vi "HFRR ADV v024 new software.vi"() -> ()   [LabVIEW 2025] (continued)
    tunnel: [w2159] -> _
    tunnel: [w2135] -> w60
    i -> [w2159]
    stop <- w2135 stop-if-true
    # "C:\\LAB-IQ-NXT\\Scar View.exe"
    n1674 = local read "OK Button 16"() -> (w2148:bool)
    n1675 = local read "Main Tab"() -> (w2141:T2)
    n1676 = local read "service 3"() -> (w2142:bool)
    n1677 = local read "OPEN 6"() -> (w2144:bool)
    n1678 = local read "EDIT 2"() -> (w2146:bool)
    n1679 = flat-sequence {
      frame #0 {
        n1680 = stacked-sequence {
          frame #0 {
            n1681 = local read "EDIT"() -> (w2813:bool)
            n1682 = case shown="True" w2813 {
              tunnel: [u8 2 ("Disabled") u8 0 ("Disabled")] -> _
              frame False {
                w2815 = FALSE
                n1683 = local write "Password"("") -> ()
                n1684 = property on="SrvM CP" class="Bool (strict)"("Visible"=w2815) -> ()  [unwired: 2 in, 2 out]
                n1685 = property on="message" class="Str"("Visible"=w2815) -> ()  [unwired: 2 in, 2 out]
                n1686 = local write "x = y?"(w2815) -> ()
                n1687 = property on="Password" class="Str"("Visible"=w2815) -> ()  [unwired: 2 in, 2 out]
                n1688 = property on="ENTER THE NEW PASSWORD" class="Str"("Visible"=w2815) -> ()  [unwired: 2 in, 2 out]
                n1689 = property on="ENTER CURRENT PASSWORD" class="Str"("Visible"=w2815) -> ()  [unwired: 2 in, 2 out]
                n1690 = local write "SrvM CP"(w2815) -> ()
              }
              frame True {
                w2818 = TRUE
                n1691 = property on="SrvM CP" class="Bool (strict)"("Visible"=w2818) -> ()  [unwired: 2 in, 2 out]
                n1692 = property on="Password" class="Str"("Visible"=w2818) -> ()  [unwired: 2 in, 2 out]
              }
            }
            "dipl pwd" <- "@143$\n" ("dipl pwd")
          }
          frame #1 {
            # "Gain password"
            n1693 = String To Byte Array(string="ENTER CURRENT PASSWORD") -> (unsigned byte array=w2823:u8[])
            n1694 = Search 1D Array(1D array=w2823, element=u8 10) -> (index of element=w2826:i32)  [unwired: 1 in]
            n1695 = Index Array(array=w2823, index=w2826) -> (element=w2822:u8)
            n1696 = Equal?(x=w2822, y=10) -> (x = y?=w2820:bool)
            n1697 = case shown="True" w2820 {
              frame False {
                n1698 = property on="ENTER THE NEW PASSWORD" class="Str"("Visible"=FALSE) -> ()  [unwired: 2 in, 2 out]
              }
              frame True {
                # "password"
                # "change password logic"
                n1699 = local read "ENTER CURRENT PASSWORD"() -> (w2839:string)
                n1700 = local read "dipl pwd"() -> (w2833:string)
                n1701 = String To Byte Array(string=w2839) -> (unsigned byte array=w2841:u8[])
                n1702 = String To Byte Array(string=w2833) -> (unsigned byte array=w2834:u8[])
                n1703 = Array Size(array=w2841) -> (size(s)=w2838:i32)
                n1704 = Array Size(array=w2834) -> (size(s)=w2836:i32)
                n1705 = for {
                  N: w2838 -> [_]
                  tunnel: w2841 -> [w2865]
                  tunnel: [w2863] -> w2842 mode=indexing
                  tunnel: w2838 -> [w2857]
                  i -> [w2858]
                  n1706 = Decrement(x=w2857) -> (x-1=w2855:i32)
                  n1707 = Equal?(x=w2858, y=w2855) -> (x = y?=w2856:bool)
                  n1708 = Index Array(array=w2865, index=w2858) -> (element=w2859:u8)
                  n1709 = Number To Decimal String(number=w2859) -> (decimal integer string=w2864:string)  [unwired: 1 in]
                  n1710 = Select(t="", s=w2856, f="\r") -> (s? t:f=w2861:string)
                  n1711 = Concatenate Strings(w2864, w2861) -> (w2863:string)
                }
                n1712 = for {
                  N: w2836 -> [_]
                  tunnel: w2834 -> [w2853]
                  tunnel: [w2851] -> w2835 mode=indexing
                  tunnel: w2836 -> [w2848]
                  i -> [w2849]
                  n1713 = Decrement(x=w2848) -> (x-1=w2847:i32)
                  n1714 = Equal?(x=w2849, y=w2847) -> (x = y?=w2846:bool)
                  n1715 = Index Array(array=w2853, index=w2849) -> (element=w2852:u8)
                  n1716 = Number To Decimal String(number=w2852) -> (decimal integer string=w2850:string)  [unwired: 1 in]
                  n1717 = Select(t="", s=w2846, f="\r") -> (s? t:f=w2843:string)
                  n1718 = Concatenate Strings(w2850, w2843) -> (w2851:string)
                }
                n1719 = local read "string"() -> (w2840:string)
                n1720 = Concatenate Strings(w2835) -> (w2829:string)
                n1721 = Concatenate Strings(w2840) -> (w2837:string)
                n1722 = Concatenate Strings(w2842) -> (w2830:string)
                n1723 = Equal?(x=w2830, y=w2837) -> (x = y?=w2832:bool)
                n1724 = Equal?(x=w2830, y=w2829) -> (x = y?=w2828:bool)
                n1725 = Or(x=w2832, y=w2828) -> (x .or. y?=w2831:bool)
                n1726 = case shown="True" w2831 {
                  frame False {
                  }
                  frame True {
                    n1727 = property on="ENTER THE NEW PASSWORD" class="Str"("Visible"=TRUE) -> ()  [unwired: 2 in, 2 out]
                  }
                }
              }
            }
          }
          frame #2 {
            n1728 = String To Byte Array(string="ENTER THE NEW PASSWORD") -> (unsigned byte array=w2868:u8[])
            n1729 = Search 1D Array(1D array=w2868, element=u8 10) -> (index of element=w2872:i32)  [unwired: 1 in]
            n1730 = Index Array(array=w2868, index=w2872) -> (element=w2870:u8)
            n1731 = Equal?(x=w2870, y=10) -> (x = y?=w2867:bool)
            n1732 = case shown="False" w2867 {
              frame False {
              }
              frame True {
                n1733 = local write "EDIT"(FALSE) -> ()
                n1734 = local write "SrvM CP"(FALSE) -> ()
                n1735 = local read "ENTER THE NEW PASSWORD"() -> (w2875:string)
                n1736 = String To Byte Array(string=w2875) -> (unsigned byte array=w2880:u8[])
                n1737 = Array Size(array=w2880) -> (size(s)=w2877:i32)
                n1738 = for {
                  N: w2877 -> [_]
                  tunnel: w2880 -> [w2893]
                  tunnel: [w2890] -> w2882 mode=indexing
                  tunnel: w2877 -> [w2885]
                  i -> [w2883]
                  n1739 = Decrement(x=w2885) -> (x-1=w2886:i32)
                  n1740 = Equal?(x=w2883, y=w2886) -> (x = y?=w2887:bool)
                  n1741 = Index Array(array=w2893, index=w2883) -> (element=w2892:u8)
                  n1742 = Number To Decimal String(number=w2892) -> (decimal integer string=w2891:string)  [unwired: 1 in]
                  n1743 = Select(t="", s=w2887, f="\r") -> (s? t:f=w2884:string)
                  n1744 = Concatenate Strings(w2891, w2884) -> (w2890:string)
                }
                n1745 = local read "file path"() -> (w2874:path)
                n1746 = Concatenate Strings(w2882) -> (w2876:string)
                n1747 = Delete(path (use dialog)=w2874) -> (deleted path=w2878:path)  [unwired: 4 in, 2 out]
                n1748 = call <vilib>:"Write Characters To File.vi"("append to file? (new file:F)"=FALSE, "character string"=w2876, "file path (dialog if empty)"=w2878) -> ()  [unwired: 2 in, 1 out]
              }
            }
          }
          frame #3 {
            n1749 = case shown="True" "SrvM CP" {
              frame False {
                w2896 = ""
                n1750 = local write "ENTER CURRENT PASSWORD"(w2896) -> ()
                n1751 = local write "ENTER THE NEW PASSWORD"(w2896) -> ()
                n1752 = property on="ENTER CURRENT PASSWORD" class="Str"("Visible"=FALSE) -> ()  [unwired: 2 in, 2 out]
              }
              frame True {
                n1753 = property on="ENTER THE NEW PASSWORD" class="Str"() -> ("Visible"=w2897:bool)  [unwired: 2 in, 2 out]
                n1754 = Not(x=w2897) -> (.not. x?=w2898:bool)
                n1755 = property on="ENTER CURRENT PASSWORD" class="Str"("Visible"=w2898) -> ()  [unwired: 2 in, 2 out]
              }
            }
          }
          frame #4 {
            n1756 = String To Byte Array(string="Password") -> (unsigned byte array=w2905:u8[])
            n1757 = Search 1D Array(1D array=w2905, element=u8 10) -> (index of element=w2903:i32)  [unwired: 1 in]
            n1758 = Index Array(array=w2905, index=w2903) -> (element=w2904:u8)
            n1759 = Equal?(x=w2904, y=10) -> (x = y?=w2900:bool)
            n1760 = case shown="True" w2900 {
              frame False {
              }
              frame True {
                # "password"
                # "password"
                n1761 = local read "Password"() -> (w2918:string)
                n1762 = String To Byte Array(string=w2918) -> (unsigned byte array=w2921:u8[])
                n1763 = String To Byte Array(string="@143$\n") -> (unsigned byte array=w2907:u8[])
                n1764 = Array Size(array=w2921) -> (size(s)=w2916:i32)
                n1765 = Array Size(array=w2907) -> (size(s)=w2912:i32)
                n1766 = for {
                  N: w2916 -> [_]
                  tunnel: w2921 -> [w2955]
                  tunnel: [w2953] -> w2922 mode=indexing
                  tunnel: w2916 -> [w2950]
                  i -> [w2951]
                  n1767 = Decrement(x=w2950) -> (x-1=w2949:i32)
                  n1768 = Index Array(array=w2955, index=w2951) -> (element=w2954:u8)
                  n1769 = Equal?(x=w2951, y=w2949) -> (x = y?=w2948:bool)
                  n1770 = Number To Decimal String(number=w2954) -> (decimal integer string=w2952:string)  [unwired: 1 in]
                  n1771 = Select(t="", s=w2948, f="\r") -> (s? t:f=w2945:string)
                  n1772 = Concatenate Strings(w2952, w2945) -> (w2953:string)
                }
                n1773 = for {
                  N: w2912 -> [_]
                  tunnel: w2907 -> [w2966]
                  tunnel: [w2964] -> w2910 mode=indexing
                  tunnel: w2912 -> [w2961]
                  i -> [w2962]
                  n1774 = Decrement(x=w2961) -> (x-1=w2960:i32)
                  n1775 = Index Array(array=w2966, index=w2962) -> (element=w2965:u8)
                  n1776 = Equal?(x=w2962, y=w2960) -> (x = y?=w2959:bool)
                  n1777 = Number To Decimal String(number=w2965) -> (decimal integer string=w2963:string)  [unwired: 1 in]
                  n1778 = Select(t="", s=w2959, f="\r") -> (s? t:f=w2956:string)
                  n1779 = Concatenate Strings(w2963, w2956) -> (w2964:string)
                }
                n1780 = local read "file path"() -> (w2906:path)
                n1781 = call <vilib>:"Read Characters From File.vi"("file path (dialog if empty)"=w2906) -> ("character string"=w2920:string)  [unwired: 5 in, 3 out]
                "string" <- w2920
                n1782 = flat-sequence {
                  tunnel: [w2923] -> w2917
                  frame #0 {
                    w2923 = ""
                    n1783 = local write "Password"(w2923) -> ()
                  }
                }
                n1784 = Concatenate Strings(w2910) -> (w2911:string)
                n1785 = Concatenate Strings(w2920) -> (w2919:string)
                n1786 = Concatenate Strings(w2922) -> (w2914:string)
                n1787 = Equal?(x=w2914, y=w2919) -> (x = y?=w2909:bool)
                n1788 = Equal?(x=w2914, y=w2911) -> (x = y?=w2915:bool)
                n1789 = Or(x=w2909, y=w2915) -> (x .or. y?=w2908:bool)
                "x = y?" <- w2908
                n1790 = case shown="True" w2908 {
                  selector: w2908 -> [w2925 _]
                  tunnel: w2917 -> [_ _]
                  frame False {
                    n1791 = And(x=w2925, y=TRUE ("Visible")) -> (x .and. y?=w2926:bool)
                    n1792 = property on="message" class="Str"("Visible"=w2926) -> ()  [unwired: 2 in, 2 out]
                  }
                  frame True {
                    n1793 = control-ref of="This VI"() -> (w2937:refnum<vi>)
                    n1794 = property class="VI"(reference=w2937) -> (reference out=w2928:refnum<vi>, error out=w2932:errorcluster, "Panel"=w2936:refnum<vi>)  [unwired: 1 in]
                    n1795 = property on="message" class="Str"("Visible"=FALSE) -> ()  [unwired: 2 in, 2 out]
                    n1796 = property class="Pnl"(reference=w2936, error in=w2932) -> (reference out=w2930:refnum<vi>, error out=w2933:errorcluster, "Panes[]"=w2935:refnum<vi>[])
                    n1797 = for {
                      tunnel: w2935 -> [w2944] mode=indexing
                      tunnel: T21."Always On" ("Horizontal Scrollbar Visibility") -> [w2943]
                      tunnel: w2933 -> [w2940]
                      tunnel: [w2939] -> w2931
                      n1798 = property class="Pane"(reference=w2944, error in=w2940, "HorizScrollbarVisibility"=w2943) -> (reference out=w2941:refnum<vi>, error out=w2942:errorcluster)
                      n1799 = Close Reference(reference=w2941, error in (no error)=w2942) -> (error out=w2939:errorcluster)
                    }
                    n1800 = Close Reference(reference=w2930, error in (no error)=w2931) -> (error out=w2929:errorcluster)
                    n1801 = Close Reference(reference=w2928, error in (no error)=w2929) -> (error out=→"error out 6":errorcluster)
                  }
                }
              }
            }
          }
        }
        n1802 = local read "x = y?"() -> (w2765:bool)
        n1803 = local read "HUMIDITY: 2"() -> (w2767:dbl)
        n1804 = local read "HUMIDITY:"() -> (w2766:dbl)
        n1805 = property on="Port 2 Error" class="Clust (strict)"("Visible"="EDIT") -> ()  [unwired: 2 in, 2 out]
        n1806 = property on="Port 1 Error" class="Clust (strict)"("Visible"="EDIT") -> ()  [unwired: 2 in, 2 out]
        n1807 = case shown="True" "SrvM CP 2" {
          frame False {
          }
          frame True {
            n1808 = local write "SrvM CP 2"(FALSE ("SrvM CP 2")) -> ()
            n1809 = local read "HUMIDITY: 2"() -> (w2806:dbl)
            n1810 = local read "TEMP INTERCEPT: 2"() -> (w2805:dbl)
            n1811 = local read "DISPLACEMENT : 4"() -> (w2809:dbl)
            n1812 = local read "TEMPERATURE : 2"() -> (w2808:dbl)
            n1813 = local read "STROKE GAIN : 2"() -> (w2810:dbl)
            n1814 = local read "FRIC. FORCE : 2"() -> (w2811:dbl)
            n1815 = local read "AIR TEMP INTERCEPT: 2"() -> (w2804:dbl)
            n1816 = local read "AIR TEMPERATURE : 2"() -> (w2807:dbl)
            n1817 = local write "HUMIDITY:"(w2806) -> ()
            n1818 = local write "AIR TEMP INTERCEPT:"(w2805) -> ()
            n1819 = local write "TEMPERATURE :"(w2808) -> ()
            n1820 = local write "FRIC. FORCE :"(w2811) -> ()
            n1821 = local write "STROKE GAIN :"(w2810) -> ()
            n1822 = local write "DISPLACEMENT :"(w2809) -> ()
            n1823 = local write "AIR TEMPERATURE :"(w2807) -> ()
            n1824 = local write "TEMP INTERCEPT:"(w2804) -> ()
          }
        }
        n1825 = And(x="EDIT", y=w2765) -> (x .and. y?=w2763:bool)
        n1826 = local read "DISPLACEMENT : 4"() -> (w2776:dbl)
        n1827 = local read "TEMPERATURE : 2"() -> (w2774:dbl)
        n1828 = local read "STROKE GAIN : 2"() -> (w2780:dbl)
        n1829 = local read "DISPLACEMENT :"() -> (w2775:dbl)
        n1830 = local read "FRIC. FORCE : 2"() -> (w2783:dbl)
        n1831 = local read "TEMPERATURE :"() -> (w2772:dbl)
        n1832 = local read "STROKE GAIN :"() -> (w2779:dbl)
        n1833 = local read "FRIC. FORCE :"() -> (w2782:dbl)
        n1834 = case shown="True" w2763 {
          tunnel: [u8 2 ("Disabled") u8 0 ("Disabled")] -> w2762
          tunnel: [w3122 TRUE ("Visible")] -> w2761
          frame False {
            w3122 = FALSE ("Visible")
            n1835 = local write "EDIT 2"(w3122) -> ()
          }
          frame True {
          }
        }
        n1836 = case shown="True" "SAVE" {
          frame False {
          }
          frame True {
            n1837 = stacked-sequence {
              seq-local: [w2976 _ _] -> [_ w3118 _]
              frame #0 {
                w2967 = 0.0 ("number")
                (unwired) i16 5 ("precision (6)")
                # "[CH1]    - FF\n[CH2]   - TEMPERATURE\n[CH3]    - Humidity\n[CH4]    - AIR TEMP\n[CH5]\\- Visa Uno\n[CH6] \\- Visa Due\n[CH7]  \\- file path\n[CH8]   - Displacement Gain\n[CHA]   - Stroke Gain\n[CHB]   - Stroke PID Gain\n[CHC]   -Language Selection\n[CHD]   -Power +\n[CHE]   -Power_\n[CHF]   -Heater\n[CHG]   -Humidity Wet\n[CHH]   -Humidity Dry\n[CHI]   -Integral Time"
                n1838 = local read "Language Selection"() -> (w3019:enum16{"English", "Russian"})
                n1839 = local read "STROKE GAIN :"() -> (w2968:dbl)
                n1840 = local read "AIR TEMPERATURE :"() -> (w2971:dbl)
                n1841 = local read "DISPLACEMENT :"() -> (w2969:dbl)
                n1842 = local read "TEMPERATURE :"() -> (w2972:dbl)
                n1843 = local read "FRIC. FORCE :"() -> (w2973:dbl)
                n1844 = local read "HUMIDITY:"() -> (w2970:dbl)
                n1845 = Path To String(path="File Path") -> (string=w3035:string)
                n1846 = Number To Fractional String(number=w2968, width (-)=i16 10 ("precision (6)"), precision (6)=i16 5) -> (F-format string=w3026:string)  [unwired: 1 in]
                n1847 = Number To Fractional String(number=w3019, width (-)=i16 10 ("precision (6)"), precision (6)=i16 5) -> (F-format string=w3015:string)  [unwired: 1 in]
                n1848 = Number To Fractional String(number=w2967, width (-)=i16 10 ("precision (6)"), precision (6)=i16 5) -> (F-format string=w3009:string)  [unwired: 1 in]
                n1849 = Number To Fractional String(number=w2967, width (-)=i16 10 ("precision (6)"), precision (6)=i16 5) -> (F-format string=w3006:string)  [unwired: 1 in]
                n1850 = Number To Fractional String(number=w2967, width (-)=i16 10 ("precision (6)"), precision (6)=i16 5) -> (F-format string=w3001:string)  [unwired: 1 in]
                n1851 = Number To Fractional String(number=w2967, width (-)=i16 10 ("precision (6)"), precision (6)=i16 5) -> (F-format string=w2998:string)  [unwired: 1 in]
                n1852 = Number To Fractional String(number=w2967, width (-)=i16 10 ("precision (6)"), precision (6)=i16 5) -> (F-format string=w2993:string)  [unwired: 1 in]
                n1853 = local read "Com Port 1"() -> (w2975:refnum<visa-resource-name>)
                n1854 = local read "Com Port 2"() -> (w2974:refnum<visa-resource-name>)
                n1855 = Concatenate Strings(w3035, "\\" ("string")) -> (w3034:string)
                n1856 = Number To Fractional String(number=w2973, width (-)=i16 10 ("precision (6)"), precision (6)=i16 5) -> (F-format string=w3067:string)  [unwired: 1 in]
                n1857 = Number To Fractional String(number=w2972, width (-)=i16 10 ("precision (6)"), precision (6)=i16 5) -> (F-format string=w3066:string)  [unwired: 1 in]
                n1858 = Number To Fractional String(number=w2970, width (-)=i16 10 ("precision (6)"), precision (6)=i16 5) -> (F-format string=w3060:string)  [unwired: 1 in]
                n1859 = Number To Fractional String(number=w2971, width (-)=i16 10 ("precision (6)"), precision (6)=i16 5) -> (F-format string=w3054:string)  [unwired: 1 in]
                n1860 = Number To Fractional String(number=w2969, width (-)=i16 10 ("precision (6)"), precision (6)=i16 5) -> (F-format string=w3027:string)  [unwired: 1 in]
                n1861 = Concatenate Strings("[CHA]" ("string"), w3026, "- Stroke Gain" ("string"), "\r") -> (w3020:string)
                n1862 = Concatenate Strings("[CHC]" ("string"), w3015, "-Language Selection" ("string"), "\r") -> (w3012:string)
                n1863 = Concatenate Strings("[CHD]" ("string"), w3009, "-Power +" ("string"), "\r") -> (w2991:string)
                n1864 = Concatenate Strings("[CHG]" ("string"), w2998, "-Humidity Wet" ("string"), "\r") -> (w2988:string)
                n1865 = Concatenate Strings("[CHH]" ("string"), w2993, "-Humidity Dry" ("string"), "\r") -> (w2987:string)
                n1866 = Concatenate Strings("[CH1]" ("string"), w3067, " - FF" ("string"), "\r") -> (w3065:string)
                n1867 = Concatenate Strings("[CH2]" ("string"), w3066, " - TEMPERATURE" ("string"), "\r") -> (w3064:string)
                n1868 = Concatenate Strings("[CH3]" ("string"), w3060, " - Humidity" ("string"), "\r") -> (w3057:string)
                n1869 = Concatenate Strings("[CH4]" ("string"), w3054, " - AIR TEMP" ("string"), "\r") -> (w3050:string)
                n1870 = Concatenate Strings("[CH5]" ("string"), w2975, "- Visa Uno" ("string"), "\r") -> (w3043:string)
                n1871 = Concatenate Strings("[CH6]" ("string"), w2974, "- Visa Due" ("string"), "\r") -> (w3038:string)
                n1872 = Concatenate Strings("[CH7]" ("string"), w3034, "- file path" ("string"), "\r") -> (w3037:string)
                n1873 = Concatenate Strings("[CH8]" ("string"), w3027, "- Displacement Gain" ("string"), "\r") -> (w3030:string)
                n1874 = Concatenate Strings("[CHE]" ("string"), w3006, "-Power_" ("string"), "\r") -> (w2990:string)
                n1875 = Concatenate Strings("[CHF]" ("string"), w3001, "-Heater" ("string"), "\r") -> (w2989:string)
                n1876 = Concatenate Strings(w3065, w3064, w3057, w3050, w3043, w3038, w3037, w3030, w3020, w3012, w2991, w2990, w2989, w2988, w2987) -> (w2976:string)
                "gain" <- w2976
              }
              frame #1 {
                n1877 = local read "Camera Port :"() -> (w3079:string)
                n1878 = local read "C3 :"() -> (w3087:refnum<visa-resource-name>)
                n1879 = local read "TEMP INTERCEPT:"() -> (w3088:dbl)
                n1880 = local read "AIR TEMP INTERCEPT:"() -> (w3089:dbl)
                n1881 = local read "Com Port 3"() -> (w3090:refnum<visa-resource-name>)
                n1882 = Concatenate Strings("[CH8]" ("string"), w3079, "- Visa Camera" ("string"), "\r") -> (w3078:string)
                n1883 = Concatenate Strings("[CH7]" ("string"), w3087, "- Visa Humidity" ("string"), "\r") -> (w3083:string)
                n1884 = Number To Fractional String(number=w3088, width (-)=i16 10 ("precision (6)"), precision (6)=i16 5) -> (F-format string=w3106:string)  [unwired: 1 in]
                n1885 = Concatenate Strings("[CHL]" ("string"), w3090, "- Visa humid" ("string"), "\r") -> (w3093:string)
                n1886 = Number To Fractional String(number=w3089, width (-)=i16 10 ("precision (6)"), precision (6)=i16 5) -> (F-format string=w3113:string)  [unwired: 1 in]
                n1887 = Concatenate Strings("[CHK]" ("string"), w3106, "-TEMP INTERCEPT" ("string"), "\r") -> (w3102:string)
                n1888 = Concatenate Strings("[SNO]" ("string"), "S.NO", "-" ("string"), "\r") -> (w3098:string)
                n1889 = Concatenate Strings("[CHJ]" ("string"), w3113, "-AIR TEMP INTERCEPT" ("string"), "\r") -> (w3103:string)
                n1890 = String To Path(string="C:\\LAB-IQ\\calibrate WO 2465.dcf") -> (path=w3091:path)
                n1891 = Concatenate Strings(w3118, w3103, w3102, w3098, w3093, w3083, w3078) -> (w3117:string)
                n1892 = call <vilib>:"Write Characters To File.vi"("append to file? (new file:F)"=FALSE, "character string"=w3117, "file path (dialog if empty)"=w3091) -> ()  [unwired: 2 in, 1 out]
              }
              frame #2 {
                n1893 = local write "Lan flag"(0.0 ("Lan flag")) -> ()
                n1894 = local write "conststatus"(0.0 ("rpm value : 2")) -> ()
                n1895 = local write "SAVE"(FALSE ("OK Button 14")) -> ()
              }
            }
          }
        }
        n1896 = Subtract(x=w2767, y=w2766) -> (x-y=w2768:dbl)
        n1897 = local read "AIR TEMPERATURE : 2"() -> (w2771:dbl)
        n1898 = local read "AIR TEMPERATURE :"() -> (w2770:dbl)
        n1899 = Divide(x=w2768, y=w2766) -> (x/y=w2790:dbl)
        n1900 = Subtract(x=w2783, y=w2782) -> (x-y=w2781:dbl)
        n1901 = Subtract(x=w2774, y=w2772) -> (x-y=w2773:dbl)
        n1902 = Subtract(x=w2780, y=w2779) -> (x-y=w2778:dbl)
        n1903 = Subtract(x=w2776, y=w2775) -> (x-y=w2777:dbl)
        n1904 = Subtract(x=w2771, y=w2770) -> (x-y=w2769:dbl)
        n1905 = Divide(x=w2781, y=w2782) -> (x/y=w2801:dbl)
        n1906 = Divide(x=w2773, y=w2772) -> (x/y=w2794:dbl)
        n1907 = Divide(x=w2778, y=w2779) -> (x/y=w2798:dbl)
        n1908 = Divide(x=w2777, y=w2775) -> (x/y=w2797:dbl)
        n1909 = Multiply(x=w2790, y=100.0) -> (x*y=→"HUMIDITY  Calibration Error":dbl)
        n1910 = Divide(x=w2769, y=w2770) -> (x/y=w2793:dbl)
        n1911 = Multiply(x=w2801, y=100.0) -> (x*y=→"FRIC. FORCE Calibration Error":dbl)
        n1912 = Multiply(x=w2794, y=100.0) -> (x*y=→"TEMPERATURE  Calibration Error":dbl)
        n1913 = Multiply(x=w2798, y=100.0) -> (x*y=→"STROKE Calibration Error":dbl)
        n1914 = Multiply(x=w2797, y=100.0) -> (x*y=→"DISPLACEMENT  Calibration Error":dbl)
        n1915 = property on="EDIT 2" class="Bool (strict)"("Visible"=w2761) -> ()  [unwired: 2 in, 2 out]
        n1916 = property on="SAVE" class="Bool (strict)"("Visible"=w2761) -> ()  [unwired: 2 in, 2 out]
        n1917 = property on="SrvM CP" class="Bool (strict)"("Disabled"=w2762) -> ()  [unwired: 2 in, 2 out]
        n1918 = property on="visa due" class="CmbBox"("Disabled"=w2762) -> ()  [unwired: 2 in, 2 out]
        n1919 = property on="File Path" class="Path"("Disabled"=w2762) -> ()  [unwired: 2 in, 2 out]
        n1920 = Multiply(x=w2793, y=100.0) -> (x*y=→"AIR TEMPERATURE  Calibration Error":dbl)
        n1921 = property on="Language Selection" class="Enum (strict)"("Visible"=w2761) -> ()  [unwired: 2 in, 2 out]
        n1922 = property on="Tab Control 7" class="TabCtl (strict)"("Disabled"=w2762) -> ()  [unwired: 2 in, 2 out]
        n1923 = property on="AIR TEMP INTERCEPT:" class="DigNum (strict)"("Disabled"=w2762) -> ()  [unwired: 2 in, 2 out]
        n1924 = property on="AIR TEMPERATURE :" class="DigNum (strict)"("Disabled"=w2762) -> ()  [unwired: 2 in, 2 out]
        n1925 = property on="STROKE GAIN :" class="DigNum (strict)"("Disabled"=w2762) -> ()  [unwired: 2 in, 2 out]
        n1926 = property on="SPEED OUT:" class="DigNum (strict)"("Disabled"=w2762) -> ()  [unwired: 2 in, 2 out]
        n1927 = property on="HUMIDITY:" class="DigNum (strict)"("Disabled"=w2762) -> ()  [unwired: 2 in, 2 out]
        n1928 = property on="TEMPERATURE :" class="DigNum (strict)"("Disabled"=w2762) -> ()  [unwired: 2 in, 2 out]
        n1929 = property on="DISPLACEMENT :" class="DigNum (strict)"("Disabled"=w2762) -> ()  [unwired: 2 in, 2 out]
        n1930 = property on="TEMP INTERCEPT:" class="DigNum (strict)"("Disabled"=w2762) -> ()  [unwired: 2 in, 2 out]
        n1931 = property on="FRIC. FORCE :" class="DigNum (strict)"("Disabled"=w2762) -> ()  [unwired: 2 in, 2 out]
      }
    }
    n1932 = local read "RUN"() -> (w2158:bool)
    n1933 = local read "RUN"() -> (w2156:bool)
    n1934 = disable-structure shown="Disabled" {
      disable-tunnel: [w2173 _] -> w2139
      disable-tunnel: [w2172 _] -> w2137
      frame Disabled {
        n1935 = local read "Temperature before test"() -> (w2166:dbl)
        n1936 = local read "Temperature after test"() -> (w2179:dbl)
        n1937 = case shown="True" "Save Results" {
          frame False {
          }
          frame True {
            w2195 = "\r"
            n1938 = local write "Save Results"(FALSE ("OK Button 5")) -> ()
            n1939 = local read "Temperature before test"() -> (w2233:dbl)
            n1940 = local read "Temperature after test"() -> (w2235:dbl)
            n1941 = local read "Humidity before test"() -> (w2232:dbl)
            n1942 = local read "Humidity after test"() -> (w2234:dbl)
            n1943 = local read "WS1.4"() -> (w2239:dbl)
            n1944 = local read "AVP"() -> (w2237:dbl)
            n1945 = Number To Fractional String(number=w2239, width (-)=i16 6, precision (6)=i16 1) -> (F-format string=w2199:string)  [unwired: 1 in]
            n1946 = local read "MWSD"() -> (w2236:dbl)
            n1947 = local read "String"() -> (w2228:string)
            n1948 = local read "FILE"() -> (w2231:string)
            n1949 = local read "HCF"() -> (w2238:dbl)
            n1950 = Number To Fractional String(number=w2232, width (-)=i16 6, precision (6)=i16 1) -> (F-format string=w2224:string)  [unwired: 1 in]
            n1951 = Number To Fractional String(number=w2233, width (-)=i16 6, precision (6)=i16 1) -> (F-format string=w2221:string)  [unwired: 1 in]
            n1952 = Number To Fractional String(number=w2234, width (-)=i16 6, precision (6)=i16 1) -> (F-format string=w2217:string)  [unwired: 1 in]
            n1953 = Number To Fractional String(number=w2235, width (-)=i16 6, precision (6)=i16 1) -> (F-format string=w2213:string)  [unwired: 1 in]
            n1954 = Number To Fractional String(number=w2237, width (-)=i16 6, precision (6)=i16 3) -> (F-format string=w2206:string)  [unwired: 1 in]
            n1955 = Concatenate Strings(w2228, w2231) -> (w2250:string)
            n1956 = Number To Fractional String(number=w2236, width (-)=i16 6, precision (6)=i16 1) -> (F-format string=w2210:string)  [unwired: 1 in]
            n1957 = Number To Fractional String(number=w2238, width (-)=i16 6, precision (6)=i16 2) -> (F-format string=w2204:string)  [unwired: 1 in]
            n1958 = Concatenate Strings("(" ("string"), w2199, ")Microns" ("string")) -> (w2198:string)
            n1959 = local read "REMARKS"() -> (w2230:string)
            "REMARKS 2" <- w2230
            n1960 = Concatenate Strings("(" ("string"), w2224, " ) % RH," ("string")) -> (w2225:string)
            n1961 = Concatenate Strings(w2204, ")" ("string")) -> (w2202:string)
            n1962 = Concatenate Strings("(" ("string"), w2221, ")  Deg C ," ("string")) -> (w2220:string)
            n1963 = Concatenate Strings("(" ("string"), w2217, " ) % RH," ("string")) -> (w2216:string)
            n1964 = Concatenate Strings("(" ("string"), w2213, ")  Deg C ," ("string")) -> (w2212:string)
            n1965 = Concatenate Strings("(" ("string"), w2210, ")  Microns," ("string")) -> (w2209:string)
            n1966 = Concatenate Strings("(" ("string"), w2206, ")  kPa," ("string")) -> (w2196:string)
            n1967 = Concatenate Strings(w2250, ".dwm" ("Substring")) -> (w2248:string)
            n1968 = String To Path(string=w2248) -> (path=w2247:path)
            n1969 = Concatenate Strings(w2230, w2195, " Humidity before test= " ("Substring"), w2225, w2195, " Temperature before test = " ("Substring"), w2220, w2195, " Humidity after test= " ("Substring"), w2216, w2195, "Temperature after test = " ("Substring"), w2212, w2195, "MSD = " ("Substring"), w2209, w2195, "  AVP = " ("Substring"), w2196, w2195, "  HCF                     =( " ("Substring"), w2202, w2195, " WS1.4                  = " ("Substring"), w2198, w2195) -> (w2194:string)
            "data" <- w2194
            n1970 = call <vilib>:"Write Characters To File.vi"("append to file? (new file:F)"=FALSE, "character string"=w2194, "file path (dialog if empty)"=w2247) -> ()  [unwired: 2 in, 1 out]
            n1971 = Match Pattern(string=w2194, regular expression="!") -> (after substring=→"export":string)  [unwired: 1 in, 3 out]
          }
        }
        n1972 = Add(x=231.864, y=w2166) -> (x+y=w2163:dbl)
        n1973 = Add(x=231.864, y=w2179) -> (x+y=w2176:dbl)
        n1974 = Divide(x=1705.984, y=w2163) -> (x/y=w2164:dbl)
        n1975 = Divide(x=1705.984, y=w2176) -> (x/y=w2177:dbl)
        n1976 = local read "Humidity before test"() -> (w2168:dbl)
        n1977 = local read "Humidity after test"() -> (w2181:dbl)
        n1978 = Subtract(x=8.017352 ("y"), y=w2164) -> (x-y=w2190:dbl)
        n1979 = Subtract(x=8.017352 ("y"), y=w2177) -> (x-y=w2184:dbl)
        n1980 = expression code="10**y"(w2190) -> (w2170:dbl)
        n1981 = expression code="10**y"(w2184) -> (w2183:dbl)
        n1982 = Multiply(x=w2168, y=w2170) -> (x*y=w2169:dbl)
        n1983 = Multiply(x=w2181, y=w2183) -> (x*y=w2182:dbl)
        n1984 = Divide(x=w2169, y=750.0) -> (x/y=w2185:dbl)
        n1985 = Divide(x=w2182, y=750.0) -> (x/y=w2186:dbl)
        n1986 = Add(x=w2185, y=w2186) -> (x+y=w2187:dbl)
        n1987 = Divide(x=w2187, y=2.0) -> (x/y=w2189:dbl)
        n1988 = local write "AVP"(w2189) -> ()
        n1989 = Subtract(x=1.4, y=w2189) -> (x-y=w2172:dbl)
        n1990 = local read "HCF"() -> (w2173:dbl)
      }
      frame Enabled {
      }
    }
    n1991 = case shown="True" "EDIT 3" {
      frame False {
      }
      frame True {
        n1992 = local write "EDIT 3"(FALSE ("EDIT 3")) -> ()
        n1993 = local write "Main Tab"(T2."About" ("Main Tab")) -> ()
      }
    }
    n1994 = case shown="False" w2158 {
      frame False {
        n1995 = local read "stopT"() -> (w3129:bool)
        n1996 = case shown="True" w3129 {
          frame False {
          }
          frame True {
            n1997 = local write "stopT"(FALSE) -> ()
          }
        }
      }
      frame True {
        "stopT" <- TRUE
      }
    }
    n1998 = case shown="False" w2156 {
      frame False {
      }
      frame True {
      }
    }
    n1999 = case shown="True" w2146 {
      frame False {
        n2000 = property on="Password 2" class="Str"("Visible"=FALSE) -> ()  [unwired: 2 in, 2 out]
        n2001 = local write "Password 2"("" ("Password")) -> ()
      }
      frame True {
        n2002 = property on="Password 2" class="Str"("Visible"=TRUE) -> ()  [unwired: 2 in, 2 out]
        n2003 = Equal?(x="Password 2", y="HFRR1234") -> (x = y?=w2278:bool)
        n2004 = case shown="True" w2278 {
          tunnel: "Password 2" -> [w2281 _]
          frame False {
            n2005 = String Length(string=w2281) -> (length=w2282:i32)
            n2006 = Greater Than 0?(x=w2282) -> (x > 0?=w2280:bool)
            n2007 = case shown="False" w2280 {
              frame False {
                n2008 = property on="Password 2" class="Str"("Caption.Text"="Password (Advance Setting)") -> ()  [unwired: 2 in, 2 out]
              }
              frame True {
                n2009 = property on="Password 2" class="Str"("Caption.Text"="Incorrect Password!") -> ()  [unwired: 2 in, 2 out]
              }
            }
          }
          frame True {
            n2010 = local write "EDIT 2"(FALSE ("EDIT 2")) -> ()
            n2011 = local write "Password 2"("" ("Password")) -> ()
            n2012 = local write "Main Tab"(T2."Advance" ("Main Tab")) -> ()
            n2013 = local write "Main Dashboard Buttons"(T1."Advance" ("Main Dashboard Buttons")) -> ()
          }
        }
      }
    }
    n2014 = case shown="True" "Prog Uno" {
      frame False {
      }
      frame True {
        n2015 = stacked-sequence {
          frame #0 {
            n2016 = Delete(path (use dialog)=path "C:/LAB-IQ-NXT/UNOCOMPILE.bat" ("working directory")) -> ()  [unwired: 4 in, 3 out]
          }
          frame #1 {
            n2017 = local read "Com Port 1"() -> (w2743:refnum<visa-resource-name>)
            n2018 = Concatenate Strings("cmd.exe /c \"mode " ("command line"), w2743, ":1200,n,8,1\"\n" ("command line")) -> (w2748:string)
            n2019 = Concatenate Strings(w2748, "CD\\\nCD WinDucom\navrdude -C avrdude.conf -v -patmega328p -carduino -P" ("command line"), w2743, " -b115200 -D -Uflash:w:UNO_V20.hex:i\n" ("command line"), "\r") -> (w2750:string)
            "STR" <- w2750
            n2020 = call <vilib>:"Write Characters To File.vi"("append to file? (new file:F)"=FALSE, "character string"=w2750, "file path (dialog if empty)"=path "C:/LAB-IQ/UNOCOMPILE.bat" ("working directory")) -> ()  [unwired: 2 in, 1 out]
          }
          frame #2 {
            n2021 = disable-structure shown="Disabled" {
              frame Disabled {
                w2754 = "cmd.exe  /c \"C:\\LAB-IQ-NXT\\UNOCOMPILE.bat\"" ("string")
                n2022 = local write "Prog Uno"(FALSE ("run minimized? (F)")) -> ()
                n2023 = call <vilib>:"System Exec.vi"("expected output size  (4096)"=u32 65535, "run minimized? (F)"=FALSE, "wait until completion? (T)"=TRUE ("run minimized? (F)"), "working directory"=path "C:/LAB-IQ-NXT", "standard input"=w2754, "command line"=w2754) -> ("error out"=w2753:errorcluster, "standard output"=→"String 42":string)  [unwired: 2 in, 2 out]
                "error out 3" <- w2753
                n2024 = flat-sequence {
                  tunnel: w2753 -> [_]
                  frame #0 {
                  }
                }
              }
              frame Enabled {
              }
            }
          }
        }
      }
    }
    n2025 = case shown="\"ISO 12156\"" "TEST STANDARD" {
      tunnel: [2.0 ("Set Temp") 0.0 ("Set Temp") 2.0 ("Set Temp") 0.0 ("Set Temp")] -> w2147
      frame "ASTM D6079", Default {
        w2700 = 50.0 ("Hz")
        w2701 = 53.0 ("Set Rh")
        w2703 = 1.0 ("Set Strk")
        w2702 = 60.0 ("Set Temp")
        # "astm hide"
        n2026 = local write "NORMAL LOAD"(200.0 ("NORMAL LOAD")) -> ()
        n2027 = local write "Set Strk"(w2703) -> ()
        n2028 = local write "Set Hz"(w2700) -> ()
        n2029 = local write "Set Temp"(w2702) -> ()
        n2030 = local write "Set Rh"(w2701) -> ()
        n2031 = local write "test time"(75.0 ("test time")) -> ()
        n2032 = local write "Set Stroke:"(w2703) -> ()
        n2033 = local write "Set Humidity:"(w2701) -> ()
        n2034 = local write "Set Frequency:"(w2700) -> ()
        n2035 = local write "Set Temperature:"(w2702) -> ()
        "Test Standard" <- "ASTM D6079" ("Test Standard 2")
      }
      frame "ISO 12156" {
        n2036 = local write "Set Strk"(1.0 ("Set Strk")) -> ()
        n2037 = local write "NORMAL LOAD"(200.0 ("NORMAL LOAD")) -> ()
        n2038 = local write "Set Temp"(60.0 ("Set Temp")) -> ()
        n2039 = local write "test time"(75.0 ("test time")) -> ()
        n2040 = local write "Set Hz"(50.0 ("Hz")) -> ()
        n2041 = local write "Set Rh"(53.0 ("Set Rh")) -> ()
      }
      frame "CEC F-096-A-06" {
        n2042 = local write "Set Strk"(1.0 ("Set Strk")) -> ()
        n2043 = local write "NORMAL LOAD"(200.0 ("NORMAL LOAD")) -> ()
        n2044 = local write "Set Temp"(60.0 ("Set Temp")) -> ()
        n2045 = local write "test time"(75.0 ("test time")) -> ()
        n2046 = local write "Set Hz"(50.0 ("Hz")) -> ()
        n2047 = local write "Set Rh"(53.0 ("Set Rh")) -> ()
      }
      frame "Custom" {
      }
    }
    n2048 = case shown="True" "Prog Due" {
      frame False {
      }
      frame True {
        n2049 = stacked-sequence {
          frame #0 {
            n2050 = Delete(path (use dialog)=path "C:/LAB-IQ/DUECOMPILE.bat" ("working directory")) -> ()  [unwired: 4 in, 3 out]
          }
          frame #1 {
            n2051 = disable-structure shown="Disabled" {
              frame Disabled {
                n2052 = local read "visa due"() -> (w2725:string)
                n2053 = Concatenate Strings("cmd.exe /c \"mode " ("command line"), w2725, ":1200,n,8,1\"\n" ("command line")) -> (w2730:string)
                n2054 = Concatenate Strings(w2730, "CD\\\nCD WinDucom\nTIMEOUT 1\n bossac.exe -i -d --port=" ("command line"), w2725, " -U false -e -w -v -b DUE.bin -R\n" ("command line"), "\r") -> (w2732:string)
                "concatenated string 2" <- w2732
                n2055 = call <vilib>:"Write Characters To File.vi"("append to file? (new file:F)"=FALSE, "character string"=w2732, "file path (dialog if empty)"=path "C:/LAB-IQ-NXT/DUECOMPILE.bat" ("working directory")) -> ()  [unwired: 2 in, 1 out]
              }
              frame Enabled {
              }
            }
          }
          frame #2 {
            # "C:\\LAB-IQ-NXT\\DUECOMPILE.bat"
            n2056 = disable-structure shown="Disabled" {
              frame Disabled {
                w2737 = "cmd.exe  /c \"C:\\LAB-IQ-NXT\\DUECOMPILE.bat\"" ("string")
                n2057 = call <vilib>:"System Exec.vi"("expected output size  (4096)"=u32 65535, "run minimized? (F)"=FALSE, "wait until completion? (T)"=TRUE ("run minimized? (F)"), "working directory"=path "C:/LAB-IQ-NXT", "standard input"=w2737, "command line"=w2737) -> ("error out"=w2736:errorcluster, "standard output"=→"String 44":string)  [unwired: 2 in, 2 out]
                "error out 4" <- w2736
                n2058 = flat-sequence {
                  tunnel: w2736 -> [_]
                  frame #0 {
                  }
                }
              }
              frame Enabled {
              }
            }
            n2059 = local write "Prog Due"(FALSE ("Prog Due")) -> ()
          }
        }
      }
    }
    n2060 = Or(x=w2144, y=w2142) -> (x .or. y?=w2143:bool)
    n2061 = case shown="\"About\"" w2141 {
      tunnel: [T27."Acquire" ("Main Tab") T27."Compare Files" ("Main Tab") T27."About" ("Main Tab")] -> w2154
      frame "Acquire", Default {
      }
      frame "Compare Files" {
      }
      frame "About" {
      }
    }
    n2062 = Or(x=w2148, y="OPEN") -> (x .or. y?=w2149:bool)
    n2063 = case shown="True" w2149 {
      tunnel: w2148 -> [_ w2289]
      frame False {
      }
      frame True {
        n2064 = stacked-sequence {
          tunnel: w2289 -> [_ w2356 _ _]
          frame #0 {
            w2305 = "  " ("String 6")
            n2065 = local write "OPEN"(FALSE ("open")) -> ()
            n2066 = local read "string1 2"() -> (w2293:string)
            n2067 = local read "string1 3"() -> (w2292:string)
            n2068 = local read "string1 4"() -> (w2291:string)
            n2069 = property on="OPEN" class="Bool (strict)"("Visible"=FALSE) -> ()  [unwired: 2 in, 2 out]
            n2070 = local write "String 6"(w2305) -> ()
            n2071 = local write "String 7"(w2305) -> ()
            n2072 = local write "String 8"(w2305) -> ()
            n2073 = local write "String 12"(w2305) -> ()
            n2074 = local read "OK Button 16"() -> (w2290:bool)
            n2075 = String To Path(string=w2293) -> (path=w2301:path)
            n2076 = String To Path(string=w2292) -> (path=w2300:path)
            n2077 = String To Path(string=w2291) -> (path=w2299:path)
            n2078 = case shown="True" w2290 {
              tunnel: [w2306 w2307] -> w2294
              frame False {
                n2079 = local read "string1"() -> (w2306:string)
              }
              frame True {
                n2080 = local read "String Indicator 4"() -> (w2307:string)
              }
            }
            n2081 = Open/Create/Replace File "Open File"(file path (use dialog)=w2301) -> (refnum out=w2297:refnum<file>)  [unwired: 5 in, 2 out]
            n2082 = Open/Create/Replace File "Open File"(file path (use dialog)=w2300) -> (refnum out=w2296:refnum<file>)  [unwired: 5 in, 2 out]
            n2083 = Open/Create/Replace File "Open File"(file path (use dialog)=w2299) -> (refnum out=w2295:refnum<file>)  [unwired: 5 in, 2 out]
            n2084 = while {
              tunnel: w2297 -> [w2319]
              i -> [w2315]
              stop <- w2314 continue-if-true
              (unwired) TRUE ("line mode (F)")
              n2085 = Read from Text File "Read File"(file (use dialog)=w2319) -> (text=w2316:string)  [unwired: 3 in, 3 out]
              n2086 = local write "Numeric 11"(w2315) -> ()
              n2087 = String Length(string=w2316) -> (length=w2318:i32)
              n2088 = Greater?(x=w2318, y=1) -> (0:w2314:bool)
            }
            n2089 = while {
              tunnel: w2296 -> [w2325]
              i -> [w2321]
              stop <- w2320 continue-if-true
              (unwired) TRUE ("line mode (F)")
              n2090 = Read from Text File "Read File"(file (use dialog)=w2325) -> (text=w2322:string)  [unwired: 3 in, 3 out]
              n2091 = local write "Numeric 12"(w2321) -> ()
              n2092 = String Length(string=w2322) -> (length=w2324:i32)
              n2093 = Greater?(x=w2324, y=1) -> (0:w2320:bool)
            }
            n2094 = while {
              tunnel: w2295 -> [w2331]
              i -> [w2327]
              stop <- w2326 continue-if-true
              (unwired) TRUE ("line mode (F)")
              n2095 = Read from Text File "Read File"(file (use dialog)=w2331) -> (text=w2328:string)  [unwired: 3 in, 3 out]
              n2096 = local write "Numeric 13"(w2327) -> ()
              n2097 = String Length(string=w2328) -> (length=w2330:i32)
              n2098 = Greater?(x=w2330, y=1) -> (0:w2326:bool)
            }
            n2099 = String To Path(string=w2294) -> (path=w2302:path)
            n2100 = Open/Create/Replace File "Open File"(file path (use dialog)=w2302) -> (refnum out=w2298:refnum<file>)  [unwired: 5 in, 2 out]
            n2101 = while {
              tunnel: w2298 -> [w2313]
              i -> [w2309]
              stop <- w2308 continue-if-true
              (unwired) TRUE ("line mode (F)")
              n2102 = Read from Text File "Read File"(file (use dialog)=w2313) -> (text=w2310:string)  [unwired: 3 in, 3 out]
              n2103 = local write "Numeric 8"(w2309) -> ()
              n2104 = String Length(string=w2310) -> (length=w2312:i32)
              n2105 = Greater?(x=w2312, y=1) -> (0:w2308:bool)
            }
          }
          frame #1 {
            w2483 = FALSE ("ACTUAL   MERGE")
            # "Sample Temp"
            # "ECR"
            # "COF"
            # "Time\nCOF\nFF\nTemp"
            n2106 = case shown="True" w2356 {
              tunnel: [w2503 w2504] -> w2357
              frame False {
                n2107 = local read "string1"() -> (w2503:string)
              }
              frame True {
                n2108 = local read "String Indicator 4"() -> (w2504:string)
              }
            }
            n2109 = local read "string1 3"() -> (w2401:string)
            n2110 = String To Path(string=w2357) -> (path=w2488:path)
            n2111 = String To Path(string=w2401) -> (path=w2499:path)
            n2112 = local read "Numeric 12"() -> (w2485:i32)
            n2113 = local read "Numeric 8"() -> (w2487:i32)
            n2114 = local read "string1 2"() -> (w2402:string)
            n2115 = local read "string1 4"() -> (w2400:string)
            n2116 = Open/Create/Replace File "Open File"(file path (use dialog)=w2488) -> (refnum out=w2502:refnum<file>, error out=w2501:errorcluster)  [unwired: 5 in, 1 out]
            n2117 = Open/Create/Replace File "Open File"(file path (use dialog)=w2499) -> (refnum out=w2495:refnum<file>, error out=w2496:errorcluster)  [unwired: 5 in, 1 out]
            n2118 = for {
              N: w2487 -> [_]
              tunnel: w2502 -> [w2650]
              tunnel: w2501 -> [w2649]
              tunnel: [w2639] -> w2414 mode=indexing
              tunnel: [w2637] -> w2471 mode=indexing
              tunnel: [w2638] -> w2466 mode=indexing
              tunnel: w2483 -> [_]
              tunnel: [w2631] -> w2468 mode=indexing
              tunnel: [w2627] -> w2437 mode=indexing
              tunnel: [w2623] -> w2412 mode=indexing
              tunnel: [w2619] -> w2393 mode=indexing
              tunnel: [w2614] -> w2353 mode=indexing
              (unwired) TRUE ("line mode (F)")
              # "freq"
              # "Stroke"
              # "Time"
              # "CoF"
              # "Humidity"
              # "Temp"
              # "Air Temp"
              # "ECR"
              n2119 = Read from Text File "Read File"(file (use dialog)=w2650, error in=w2649) -> (text=w2615:string)  [unwired: 2 in, 3 out]
              n2120 = local write "String 6"(w2615) -> ()
              n2121 = String Subset(string=w2615, offset (0)=0, length (rest)=14 ("length (rest)")) -> (substring=w2643:string)
              n2122 = String Subset(string=w2615, offset (0)=35, length (rest)=9 ("length (rest)")) -> (substring=w2640:string)
              n2123 = String Subset(string=w2615, offset (0)=15, length (rest)=9 ("length (rest)")) -> (substring=w2646:string)
              n2124 = Fract/Exp String To Number(string=w2643) -> (number=w2639:dbl)  [unwired: 3 in, 1 out]
              n2125 = Fract/Exp String To Number(string=w2640) -> (number=w2638:dbl)  [unwired: 3 in, 1 out]
              n2126 = Fract/Exp String To Number(string=w2646) -> (number=w2637:dbl)  [unwired: 3 in, 1 out]
              n2127 = String Subset(string=w2615, offset (0)=85, length (rest)=9 ("length (rest)")) -> (substring=w2616:string)
              n2128 = String Subset(string=w2615, offset (0)=25, length (rest)=9 ("length (rest)")) -> (substring=w2622:string)
              n2129 = String Subset(string=w2615, offset (0)=55, length (rest)=9 ("length (rest)")) -> (substring=w2624:string)
              n2130 = String Subset(string=w2615, offset (0)=45, length (rest)=9 ("length (rest)")) -> (substring=w2630:string)
              n2131 = String Subset(string=w2615, offset (0)=65, length (rest)=9 ("length (rest)")) -> (substring=w2636:string)
              n2132 = Fract/Exp String To Number(string=w2622) -> (number=w2619:dbl)  [unwired: 3 in, 1 out]
              n2133 = Fract/Exp String To Number(string=w2616) -> (number=w2614:dbl)  [unwired: 3 in, 1 out]
              n2134 = Fract/Exp String To Number(string=w2624) -> (number=w2623:dbl)  [unwired: 3 in, 1 out]
              n2135 = Fract/Exp String To Number(string=w2630) -> (number=w2627:dbl)  [unwired: 3 in, 1 out]
              n2136 = Fract/Exp String To Number(string=w2636) -> (number=w2633:dbl)  [unwired: 3 in, 1 out]
              n2137 = Add(x=w2633, y=0.0) -> (x+y=w2631:dbl)
            }
            n2138 = for {
              N: w2485 -> [_]
              tunnel: w2496 -> [w2576]
              tunnel: w2495 -> [w2575]
              tunnel: [w2565] -> w2454 mode=indexing
              tunnel: [w2563] -> w2452 mode=indexing
              tunnel: [w2564] -> w2448 mode=indexing
              tunnel: w2483 -> [_]
              tunnel: [w2557] -> w2450 mode=indexing
              tunnel: [w2553] -> w2432 mode=indexing
              tunnel: [w2549] -> w2408 mode=indexing
              tunnel: [w2546] -> w2389 mode=indexing
              tunnel: [w2542] -> w2348 mode=indexing
              (unwired) 9 ("length (rest)")
              (unwired) 9 ("length (rest)")
              (unwired) TRUE ("line mode (F)")
              n2139 = Read from Text File "Read File"(file (use dialog)=w2575, error in=w2576) -> (text=w2543:string)  [unwired: 2 in, 3 out]
              n2140 = local write "String 8"(w2543) -> ()
              n2141 = String Subset(string=w2543, offset (0)=85) -> (substring=w2545:string)  [unwired: 1 in]
              n2142 = String Subset(string=w2543, offset (0)=35, length (rest)=9 ("length (rest)")) -> (substring=w2566:string)
              n2143 = String Subset(string=w2543, offset (0)=55, length (rest)=9 ("length (rest)")) -> (substring=w2551:string)
              n2144 = String Subset(string=w2543, offset (0)=25) -> (substring=w2547:string)  [unwired: 1 in]
              n2145 = String Subset(string=w2543, offset (0)=15, length (rest)=9 ("length (rest)")) -> (substring=w2572:string)
              n2146 = String Subset(string=w2543, offset (0)=0, length (rest)=14 ("length (rest)")) -> (substring=w2569:string)
              n2147 = String Subset(string=w2543, offset (0)=45, length (rest)=9 ("length (rest)")) -> (substring=w2556:string)
              n2148 = String Subset(string=w2543, offset (0)=65, length (rest)=9 ("length (rest)")) -> (substring=w2562:string)
              n2149 = Fract/Exp String To Number(string=w2545) -> (number=w2542:dbl)  [unwired: 3 in, 1 out]
              n2150 = Fract/Exp String To Number(string=w2566) -> (number=w2564:dbl)  [unwired: 3 in, 1 out]
              n2151 = Fract/Exp String To Number(string=w2551) -> (number=w2549:dbl)  [unwired: 3 in, 1 out]
              n2152 = Fract/Exp String To Number(string=w2547) -> (number=w2546:dbl)  [unwired: 3 in, 1 out]
              n2153 = Fract/Exp String To Number(string=w2572) -> (number=w2563:dbl)  [unwired: 3 in, 1 out]
              n2154 = Fract/Exp String To Number(string=w2569) -> (number=w2565:dbl)  [unwired: 3 in, 1 out]
              n2155 = Fract/Exp String To Number(string=w2556) -> (number=w2553:dbl)  [unwired: 3 in, 1 out]
              n2156 = Fract/Exp String To Number(string=w2562) -> (number=w2559:dbl)  [unwired: 3 in, 1 out]
              n2157 = Add(x=w2559, y=0.0) -> (x+y=w2557:dbl)
            }
            n2158 = String To Path(string=w2402) -> (path=w2500:path)
            n2159 = String To Path(string=w2400) -> (path=w2494:path)
            n2160 = local read "Numeric 11"() -> (w2484:i32)
            n2161 = local read "Numeric 13"() -> (w2486:i32)
            n2162 = Open/Create/Replace File "Open File"(file path (use dialog)=w2500) -> (refnum out=w2498:refnum<file>, error out=w2497:errorcluster)  [unwired: 5 in, 1 out]
            n2163 = Open/Create/Replace File "Open File"(file path (use dialog)=w2494) -> (refnum out=w2493:refnum<file>, error out=w2492:errorcluster)  [unwired: 5 in, 1 out]
            n2164 = for {
              N: w2484 -> [_]
              tunnel: w2498 -> [w2613]
              tunnel: w2497 -> [w2612]
              tunnel: [w2602] -> w2464 mode=indexing
              tunnel: [w2600] -> w2462 mode=indexing
              tunnel: [w2601] -> w2457 mode=indexing
              tunnel: w2483 -> [_]
              tunnel: [w2594] -> w2459 mode=indexing
              tunnel: [w2590] -> w2435 mode=indexing
              tunnel: [w2586] -> w2410 mode=indexing
              tunnel: [w2582] -> w2391 mode=indexing
              tunnel: [w2577] -> w2349 mode=indexing
              (unwired) TRUE ("line mode (F)")
              n2165 = Read from Text File "Read File"(file (use dialog)=w2613, error in=w2612) -> (text=w2578:string)  [unwired: 2 in, 3 out]
              n2166 = local write "String 7"(w2578) -> ()
              n2167 = String Subset(string=w2578, offset (0)=85, length (rest)=9 ("length (rest)")) -> (substring=w2581:string)
              n2168 = String Subset(string=w2578, offset (0)=35, length (rest)=9 ("length (rest)")) -> (substring=w2603:string)
              n2169 = String Subset(string=w2578, offset (0)=55, length (rest)=9 ("length (rest)")) -> (substring=w2589:string)
              n2170 = String Subset(string=w2578, offset (0)=25, length (rest)=9 ("length (rest)")) -> (substring=w2583:string)
              n2171 = String Subset(string=w2578, offset (0)=45, length (rest)=9 ("length (rest)")) -> (substring=w2591:string)
              n2172 = String Subset(string=w2578, offset (0)=0, length (rest)=14 ("length (rest)")) -> (substring=w2606:string)
              n2173 = String Subset(string=w2578, offset (0)=15, length (rest)=9 ("length (rest)")) -> (substring=w2609:string)
              n2174 = String Subset(string=w2578, offset (0)=65, length (rest)=9 ("length (rest)")) -> (substring=w2595:string)
              n2175 = Fract/Exp String To Number(string=w2581) -> (number=w2577:dbl)  [unwired: 3 in, 1 out]
              n2176 = Fract/Exp String To Number(string=w2603) -> (number=w2601:dbl)  [unwired: 3 in, 1 out]
              n2177 = Fract/Exp String To Number(string=w2589) -> (number=w2586:dbl)  [unwired: 3 in, 1 out]
              n2178 = Fract/Exp String To Number(string=w2583) -> (number=w2582:dbl)  [unwired: 3 in, 1 out]
              n2179 = Fract/Exp String To Number(string=w2591) -> (number=w2590:dbl)  [unwired: 3 in, 1 out]
              n2180 = Fract/Exp String To Number(string=w2606) -> (number=w2602:dbl)  [unwired: 3 in, 1 out]
              n2181 = Fract/Exp String To Number(string=w2609) -> (number=w2600:dbl)  [unwired: 3 in, 1 out]
